vi "Schedule Auto Calibration.vi"(6 "Start Time":u32 max=23 step=1, 8 "error in (no error)":errorcluster, 9 "Schedule Interval":u16(ring) items=["Every 8 hours", "Every 16 hours", "Every day", "Every 7 days", "Every 14 days", "Every 30 days", "Every 90 days"], 10 "Action":u16(ring) items=["Run ", "Notify", "None"], 11 "VISA resource name":refnum<visa-resource-name>) -> (0 "error out":errorcluster, 3 "VISA resource name out":refnum<visa-resource-name>)   [LabVIEW 2009, in "Keithley DMM7510.lvlib"]
doc: "This VI schedules how often auto calibration occurs or prompts/notify you to run it."
uses:
  Keithley DMM7510.lvlib
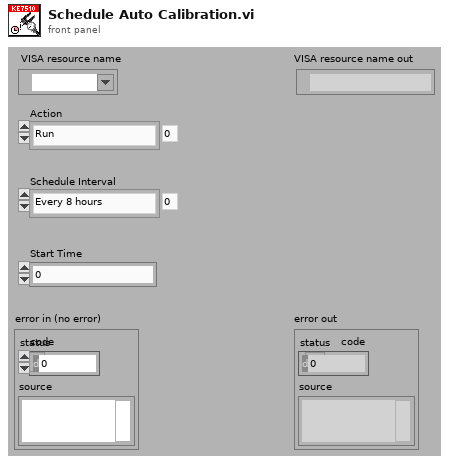
[diagram p1: front panel]
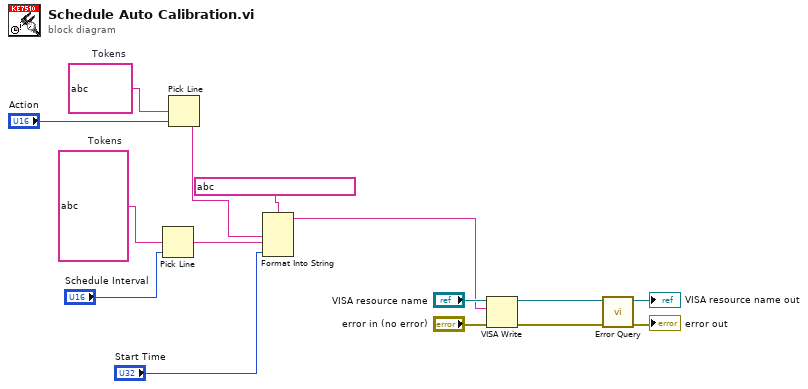
[diagram p0: block diagram]
diagram:
  w5 = string ?  # Tokens
  w8 = string ?  # Tokens
  n1 = Pick Line(multi-line string=w5, line index="Schedule Interval") -> (output string=w4:string)  [unwired: 1 out]
  n2 = Pick Line(multi-line string=w8, line index="Action") -> (output string=w3:string)  [unwired: 1 out]
  n3 = Format Into String(format string=string ?, w3, w4, "Start Time") -> (resulting string=w1:string)  [unwired: 2 in, 1 out]
  n4 = VISA Write(VISA resource name="VISA resource name", write buffer=w1, error in (no error)="error in (no error)") -> (VISA resource name out=w11:refnum<visa-resource-name>, error out=w10:errorcluster)  [unwired: 1 out]
  n5 = call "Error Query.vi"("error in (no error)"=w10, "VISA resource name"=w11) -> ("error out"=→"error out":errorcluster, "VISA resource name out"=→"VISA resource name out":refnum<visa-resource-name>)  [unwired: 6 in, 2 out]
